vi "Tests.vi"   [LabVIEW 2018]
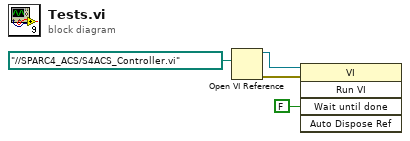
[diagram p0: block diagram]
diagram:
  n1 = Open VI Reference(vi path=path "../../SPARC4_ACS/S4ACS_Controller.vi") -> (vi reference=w4:refnum<vi>, error out=w3:errorcluster)  [unwired: 5 in]
  n2 = invoke class="VI" method="Run VI"(reference=w4, error in=w3, "Wait until done"=FALSE ("Wait Until Done")) -> ()  [unwired: 2 in, 5 out]
